vi "Init Assert Data Message.vi"(5 "Assert Data Message":refnum<class "TestManagerMsg.Assertion.lvclass">, 7 "overwrite?":bool=TRUE, 9 "Assert Data":T1={"Label"="", "Asserted"=FALSE, "call-chain"=[], "upstream-error"={"status"=FALSE, "code"=0, "source"=""}, "timestamp"=timestamp(0 s since 1904-01-01), "Execution time (s)"=-1.0}, 10 "AssertID":string, 11 "TestID":string) -> (3 "Message":refnum<class "TestManagerMsg.lvclass">)   [LabVIEW 2020, in "Caraya.lvlib" / "TestManagerMsg.Assertion.lvclass"]
uses:
  TestManagerMsg.Assertion.lvclass
  C:/projects/caraya/src/classes/Test Manager Message/TestManagerMsg.lvclass
  Test Manager Message/TestManagerMsg.lvclass
  Assert-Data -- cluster.ctl
  TestManagerMsg.Assertion.lvclass/TestManagerMsg.Assertion.ctl
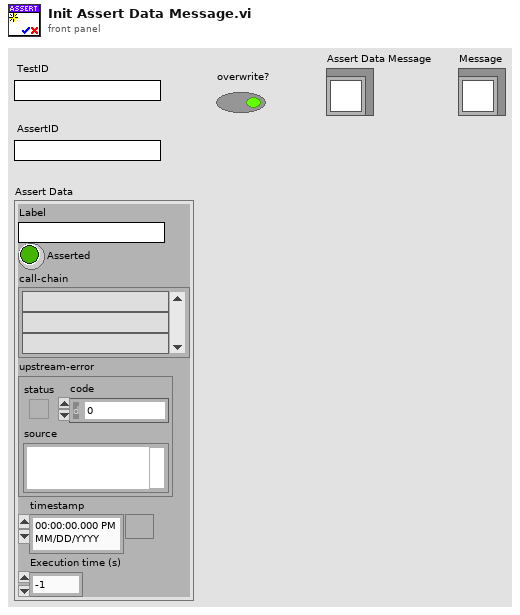
[diagram p1: front panel]
types:
  T1 = typedef "Caraya.lvlib/TestManagerMsg.Assertion.lvclass/Assert-Data -- cluster.ctl" = cluster{"Label":string, "Asserted":bool, "call-chain":string[], "upstream-error":errorcluster, "timestamp":timestamp, "Execution time (s)":dbl}
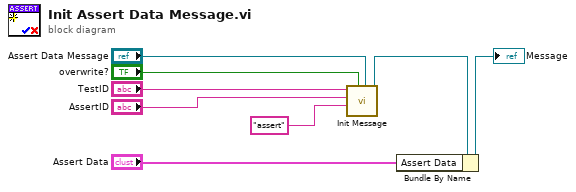
[diagram p0: block diagram]
diagram:
  n1 = call "Init Message.vi"("TestManagerMsg"="Assert Data Message", "overwrite?"="overwrite?", "key"="assert", "self-id"="AssertID", "owner-id"="TestID") -> ("Message"=w7:refnum<class "TestManagerMsg.Assertion.lvclass">)  [unwired: 6 in]
  n2 = Bundle By Name(cluster=w7, "Assert Data"="Assert Data") -> (→"Message":refnum<class "TestManagerMsg.Assertion.lvclass">)
